vi "test array manipulation.vi"() -> ()   [LabVIEW 2021]
panel:
  out "array w/ subset deleted":dbl[](array[numeric])
  in  "idx":i32
  in  "Array":dbl[](array[numeric])
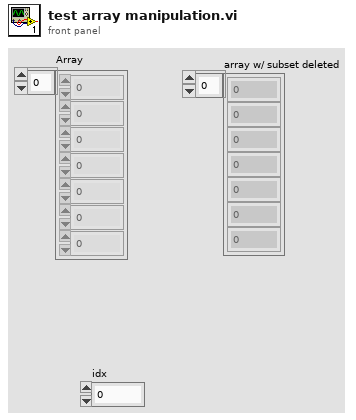
[diagram p1: front panel]
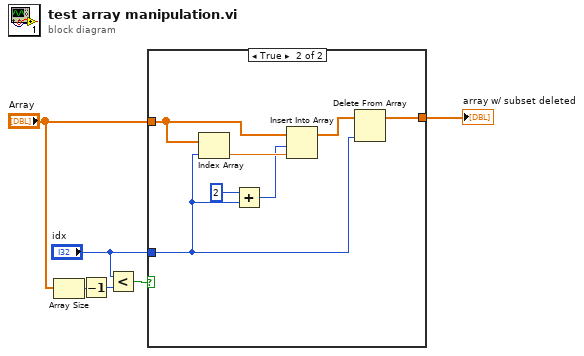
[diagram p0: block diagram]
diagram:
  n1 = Array Size(array="Array") -> (size(s)=w4:i32)
  n2 = Decrement(x=w4) -> (x-1=w2:i32)
  n3 = Less?(x="idx", y=w2) -> (x < y?=w1:bool)
  n4 = case shown="True" w1 {
    tunnel: [w7 w11] -> w6
    tunnel: "Array" -> [w7 w9]
    tunnel: "idx" -> [_ w8]
    frame False {
    }
    frame True {
      n5 = Index Array(array=w9, index=w8) -> (element=w14:dbl)
      n6 = Add(x=2, y=w8) -> (x+y=w12:i32)
      n7 = Insert Into Array(array=w9, index=w12, new element=w14) -> (w13:dbl[])
      n8 = Delete From Array(array=w13, index=w8) -> (array with subset deleted=w11:dbl[])  [unwired: 1 in, 1 out]
    }
  }
  "array w/ subset deleted" <- w6
